vi "Add New Message.vi"(8 "error in (no error)":errorcluster, 11 "Node Ptr":u64 format="%.0x") -> (0 "error out":errorcluster)   [LabVIEW 2019, in "Instrument Addon System Explorer.lvlib"]
uses:
  Instrument Addon System Explorer.lvlib
  <vilib>/NI VeriStand/Custom Device API/Custom Device API.lvlib
  <vilib>/NI VeriStand/Custom Device API/Custom Device Channel Type.ctl
  <vilib>/NI VeriStand/Custom Device API/Custom Device Channel.ctl
  Addon Shared/SubVIs/Constants.vi
  Addon Shared/Instrument Addon Shared.lvlib
  <vilib>/NI VeriStand/Custom Device Tools/Custom Device Utility Library/Search Direction.ctl
  <vilib>/NI VeriStand/Custom Device Tools/Custom Device Utility Library/Custom Device Utility Library.lvlib
  <vilib>/NI VeriStand/Custom Device Tools/Custom Device Utility Library/NI VeriStand - Search for Item by GUID.vi
panel:
  in  "Tag":string
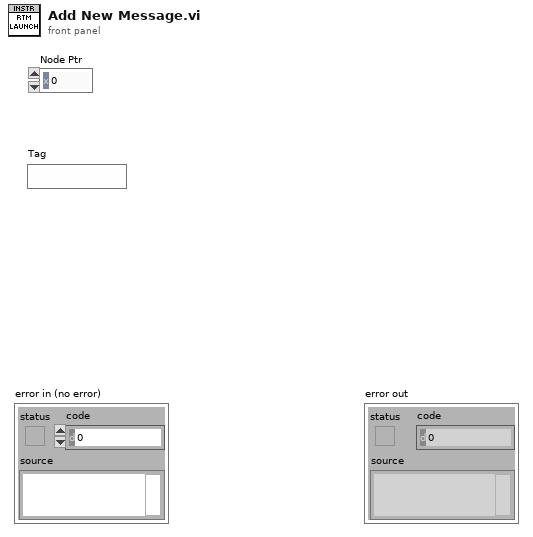
[diagram p1: front panel]
types:
  T1 = typedef "Custom Device API.lvlib/Custom Device Channel.ctl" = cluster{"Type":T2, "Units":string, "Default Value":dbl, "Faultable":bool, "Scalable":bool}
  T2 = typedef "Custom Device API.lvlib/Custom Device Channel Type.ctl" = enum16{"Input", "Output"}
  T3 = typedef "Custom Device Utility Library.lvlib/Search Direction.ctl" = enum16{"Down", "Up"}
  T4 = typedef "Custom Device API.lvlib/Custom Device Item Ref.ctl" = u64
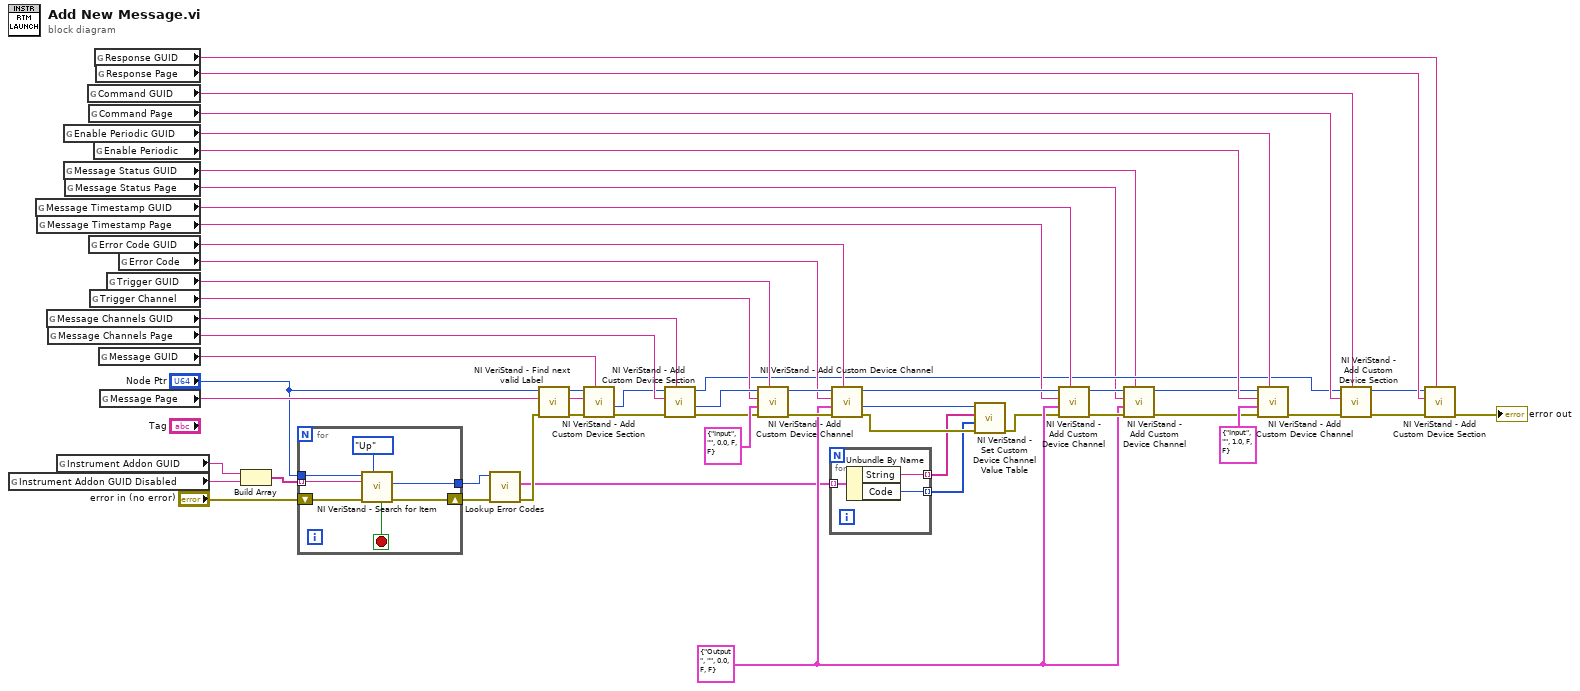
[diagram p0: block diagram]
diagram:
  w19 = T1 {"Type"=enum."Output", "Units"="", "Default Value"=0.0, "Faultable"=FALSE, "Scalable"=FALSE} ("Channel")
  n1 = global read "Constants.vi" "Instrument Addon GUID Disabled"() -> (w7:string)
  n2 = global read "Constants.vi" "Message Timestamp GUID"() -> (w31:string)
  n3 = global read "Constants.vi" "Message Timestamp Page"() -> (w30:string)
  n4 = global read "Constants.vi" "Message Channels GUID"() -> (w47:string)
  n5 = global read "Constants.vi" "Message Channels Page"() -> (w48:string)
  n6 = global read "Constants.vi" "Instrument Addon GUID"() -> (w5:string)
  n7 = global read "Constants.vi" "Enable Periodic GUID"() -> (w29:string)
  n8 = global read "Constants.vi" "Message Status GUID"() -> (w16:string)
  n9 = global read "Constants.vi" "Message Status Page"() -> (w15:string)
  n10 = global read "Constants.vi" "Command GUID"() -> (w36:string)
  n11 = global read "Constants.vi" "Command Page"() -> (w35:string)
  n12 = global read "Constants.vi" "Error Code GUID"() -> (w40:string)
  n13 = global read "Constants.vi" "Trigger Channel"() -> (w43:string)
  n14 = global read "Constants.vi" "Enable Periodic"() -> (w28:string)
  n15 = global read "Constants.vi" "Response GUID"() -> (w37:string)
  n16 = global read "Constants.vi" "Response Page"() -> (w38:string)
  n17 = global read "Constants.vi" "Message GUID"() -> (w49:string)
  n18 = global read "Constants.vi" "Message Page"() -> (w50:string)
  n19 = global read "Constants.vi" "Trigger GUID"() -> (w44:string)
  n20 = global read "Constants.vi" "Error Code"() -> (w39:string)
  n21 = Build Array(w5, w7) -> (w6:string[])
  n22 = for {
    tunnel: w6 -> [w59] mode=indexing
    tunnel: [w57] -> w1
    shift-right: [w56] -> w3
    shift-left: "error in (no error)" -> [w60]
    tunnel: "Node Ptr" -> [w55]
    stop <- w58 stop-if-true
    n23 = call-poly <vilib>:"NI VeriStand - Search for Item.vi"("Direction (Down)"=Search_Direction."Up", "error in"=w60, "Item GUID"=w59, "Section Ref in"=w55) -> ("error out"=w56:errorcluster, "Item Ref"=w57:T4, "Found"=w58:bool)  [unwired: 4 in, 1 out]
  }
  n24 = call "Lookup Error Codes.vi"("error in (no error)"=w3, "Node Ptr"=w1) -> ("error out"=w14:errorcluster, "Error Codes"=w10:cluster{"Code":i32, "String":string}[])  [unwired: 7 in, 1 out]
  n25 = call <vilib>:"NI VeriStand - Find next valid Label.vi"("error in (no error)"=w14, "Label"=w50, "Item Ref in"="Node Ptr") -> ("error out"=w53:errorcluster, "Label out"=w52:string, "Item Ref out"=w51:T4)  [unwired: 4 in, 2 out]
  n26 = call <vilib>:"NI VeriStand - Add Custom Device Section.vi"("GUID (Default Section)"=w49, "error in (no error)"=w53, "Section Name"=w52, "Parent Ref in"=w51) -> ("error out"=w24:errorcluster, "Section Ptr"=w23:T4)  [unwired: 4 in, 2 out]
  n27 = call <vilib>:"NI VeriStand - Add Custom Device Section.vi"("GUID (Default Section)"=w47, "error in (no error)"=w24, "Section Name"=w48, "Parent Ref in"=w23) -> ("error out"=w46:errorcluster, "Section Ptr"=w45:T4, "Parent Ref out"=w22:T4)  [unwired: 4 in, 1 out]
  n28 = call <vilib>:"NI VeriStand - Add Custom Device Channel.vi"("GUID (Default Channel)"=w44, "error in (no error)"=w46, "Channel"=T1 {"Type"=enum."Input", "Units"="", "Default Value"=0.0, "Faultable"=FALSE, "Scalable"=FALSE}, "Channel Name"=w43, "Parent Ref in"=w45) -> ("error out"=w42:errorcluster, "Parent Ref out"=w41:T4)  [unwired: 3 in, 2 out]
  n29 = for {
    tunnel: w10 -> [w64] mode=indexing
    tunnel: [w63] -> w8 mode=indexing
    tunnel: [w62] -> w9 mode=indexing
    n30 = Unbundle By Name(w64) -> ("String"=w63:string, "Code"=w62:i32)
  }
  n31 = call <vilib>:"NI VeriStand - Add Custom Device Channel.vi"("GUID (Default Channel)"=w40, "error in (no error)"=w42, "Channel"=w19, "Channel Name"=w39, "Parent Ref in"=w41) -> ("error out"=w12:errorcluster, "Channel Ref"=w13:T4, "Parent Ref out"=w32:T4)  [unwired: 3 in, 1 out]
  n32 = call <vilib>:"NI VeriStand - Set Custom Device Channel Value Table.vi"("error in (no error)"=w12, "Values"=w9, "Names"=w8, "Channel Ref in"=w13) -> ("error out"=w11:errorcluster)  [unwired: 6 in, 1 out]
  n33 = call <vilib>:"NI VeriStand - Add Custom Device Channel.vi"("GUID (Default Channel)"=w31, "error in (no error)"=w11, "Channel"=w19, "Channel Name"=w30, "Parent Ref in"=w32) -> ("error out"=w21:errorcluster, "Parent Ref out"=w20:T4)  [unwired: 3 in, 2 out]
  n34 = call <vilib>:"NI VeriStand - Add Custom Device Channel.vi"("GUID (Default Channel)"=w16, "error in (no error)"=w21, "Channel"=w19, "Channel Name"=w15, "Parent Ref in"=w20) -> ("error out"=w18:errorcluster, "Parent Ref out"=w17:T4)  [unwired: 3 in, 2 out]
  n35 = call <vilib>:"NI VeriStand - Add Custom Device Channel.vi"("GUID (Default Channel)"=w29, "error in (no error)"=w18, "Channel"=T1 {"Type"=enum."Input", "Units"="", "Default Value"=1.0, "Faultable"=FALSE, "Scalable"=FALSE}, "Channel Name"=w28, "Parent Ref in"=w17) -> ("error out"=w26:errorcluster)  [unwired: 3 in, 3 out]
  n36 = call <vilib>:"NI VeriStand - Add Custom Device Section.vi"("GUID (Default Section)"=w36, "error in (no error)"=w26, "Section Name"=w35, "Parent Ref in"=w22) -> ("error out"=w34:errorcluster, "Parent Ref out"=w33:T4)  [unwired: 4 in, 2 out]
  n37 = call <vilib>:"NI VeriStand - Add Custom Device Section.vi"("GUID (Default Section)"=w37, "error in (no error)"=w34, "Section Name"=w38, "Parent Ref in"=w33) -> ("error out"=→"error out":errorcluster)  [unwired: 4 in, 3 out]
